vi "RSZVB Set Mixer Delay Aperture.vi"(8 "error in (no error)":errorcluster {"code" format="%.0x"}, 9 "Aperture (0.0 Hz)":dbl format="%^.3e", 10 "Channel (1)":i32=1, 11 "VISA session":refnum<visa-resource-name>) -> (0 "error out":errorcluster {"code" format="%.0x"}, 3 "dup VISA session":refnum<visa-resource-name>)   [LabVIEW 2011]
doc: "Sets the frequency difference between the upper and lower tone (aperture). \n\nNotes:\n\n(1) This VI requires options R&S ZVA-K9, R&S ZVA-K4 and ZVT20-B11.\n\nRemote-control command(s):\n[SENSe<Ch>:]FREQuency:MDELay:APERture"
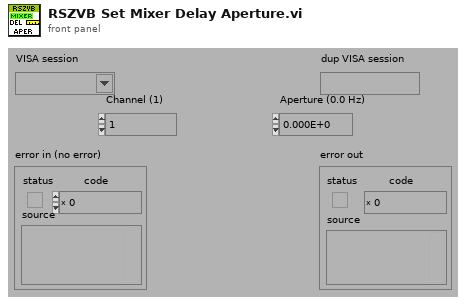
[diagram p1: front panel]
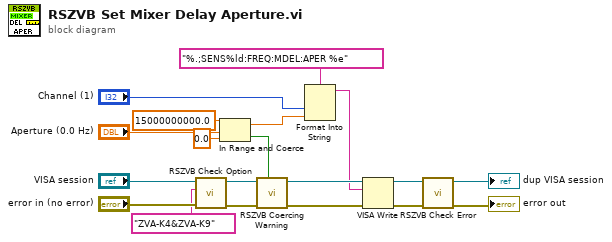
[diagram p0: block diagram]
diagram:
  n1 = call "RSZVB Check Option.vi"("error in (no error)"="error in (no error)", "Options"="ZVA-K4&ZVA-K9", "VISA session"="VISA session") -> ("error out"=w12:errorcluster, "dup VISA session"=w11:refnum<visa-resource-name>)  [unwired: 7 in]
  n2 = In Range and Coerce(upper limit=15000000000.0, x="Aperture (0.0 Hz)", lower limit=0.0) -> (coerced(x)=w8:dbl, In Range?=w13:bool)
  n3 = call "RSZVB Coercing Warning.vi"("In Range?"=w13, "error in (no error)"=w12, "VISA session"=w11) -> ("error out"=w7:errorcluster, "dup VISA session"=w6:refnum<visa-resource-name>)  [unwired: 7 in]
  n4 = Format Into String(format string="%.;SENS%ld:FREQ:MDEL:APER %e", "Channel (1)", w8) -> (resulting string=w5:string)  [unwired: 2 in, 1 out]
  n5 = VISA Write(VISA resource name=w6, write buffer=w5, error in (no error)=w7) -> (VISA resource name out=w3:refnum<visa-resource-name>, error out=w4:errorcluster)  [unwired: 1 out]
  n6 = call "RSZVB Check Error.vi"("error in (no error)"=w4, "VISA session"=w3) -> ("error out"=→"error out":errorcluster, "dup VISA session"=→"dup VISA session":refnum<visa-resource-name>)  [unwired: 8 in]
